vi "Circulos.vi"() -> ()   [LabVIEW 2014]
doc: "Newport Motion Controler\nThis VI test a Group\n\nAndré Romero - 2022\nandretec@ifsc.usp.br"
uses:
  <vilib>/Platform/TimedLoop/XDataNode/timing_clust.ctl
  <vilib>/Platform/TimedLoop/XDataNode/nitl_modes.ctl
  <vilib>/Platform/TimedLoop/XDataNode/wakeup.ctl
  <vilib>/Platform/TimedLoop/XDataNode/XDataNode.xnode
  <userlib>/Newport ESP301/Newport ESP301.lvlib
  <vilib>/Platform/TimedLoop/XDataNode/XDNodeRunTimeDep.lvlib
panel:
  in  "Decceleration (mm/s²)":dbl min=0.0 format="%.6g"
  in  "Acceleration (mm/s²)":dbl min=0.0 format="%.6g"
  in  "coordenada x_centro":dbl format="%#_13g"
  in  "arc sweep angle":dbl=-46.7 format="%#_13g"
  in  "coordenada y_centro":dbl=-5.5 format="%#_13g"
  in  "Stop Button":bool
  out "error out":errorcluster
  out "Y":dbl format="%.2g"
  out "X":dbl=1.0 format="%.2f"
  out "XY Graph":cluster{dbl[], dbl[]}(graph)
  in  "Velocity (mm/s)":dbl=0.05
  # "1o arco"
  # "2o arco"
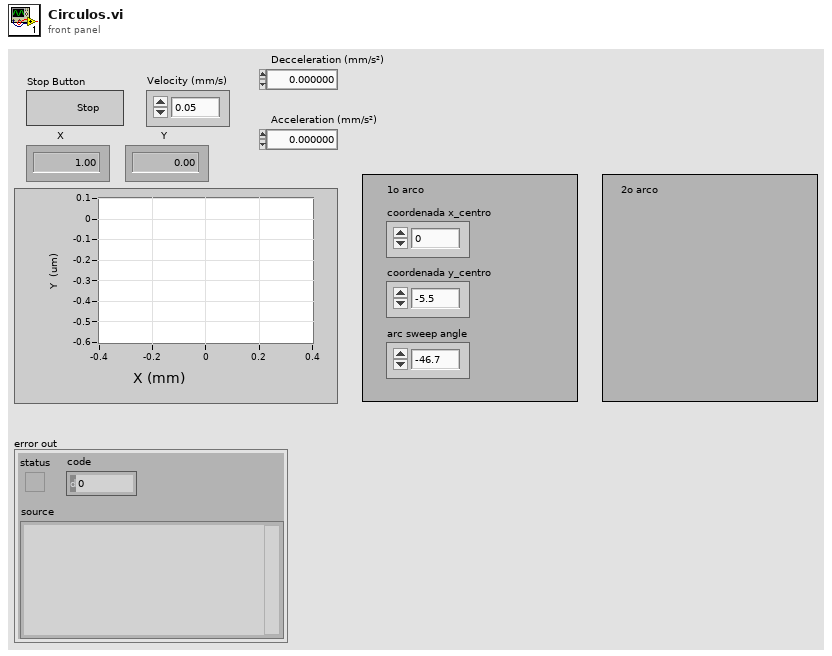
[diagram p1: front panel]
types:
  T1 = typedef "XDNodeRunTimeDep.lvlib/timing_clust.ctl" = cluster{"Expected End [f-1]":u64, "Actual End [f-1]":u64, "Finished Late? [f-1]":bool, "Expected End [i-1]":u64, "Actual End [i-1]":u64, "Finished Late? [i-1]":bool, "Expected Start [i]":u64, "Actual Start [i]":u64, "Expected Start [f]":u64, "Actual Start [f]":u64, "Source Name":string, "Structure Name":string, "Period":i64, "Deadline":i64, "Offset":i64, "Start":i64, "Priority":i32, "Timeout":i32, "Mode":T2, "Wakeup Reason":T3, "Error":errorcluster, "Source Type":string, "Secondary Source Type":string, "Global End Time":u64, "Global Start Time":u64, "Frame Duration":u64, "Iteration Duration":u64, "Assigned CPU":i32, "I/O Scan Engine Mode":u32}
  T2 = typedef "XDNodeRunTimeDep.lvlib/nitl_modes.ctl" = enum32{"No Change", "Process missed periods, maintain original phase", "Discard missed periods, maintain original phase", "Process missed periods, ignore original phase", "Discard missed periods, ignore original phase"}
  T3 = typedef "XDNodeRunTimeDep.lvlib/wakeup.ctl" = enum32{"Normal", "Aborted", "Asynchronous wakeup", "Timing source error", "Timed loop error", "Timeout"}
  T4 = cluster{"coordenada x_centro":dbl, "coordenada y_centro":dbl, "arc sweep angle":dbl}
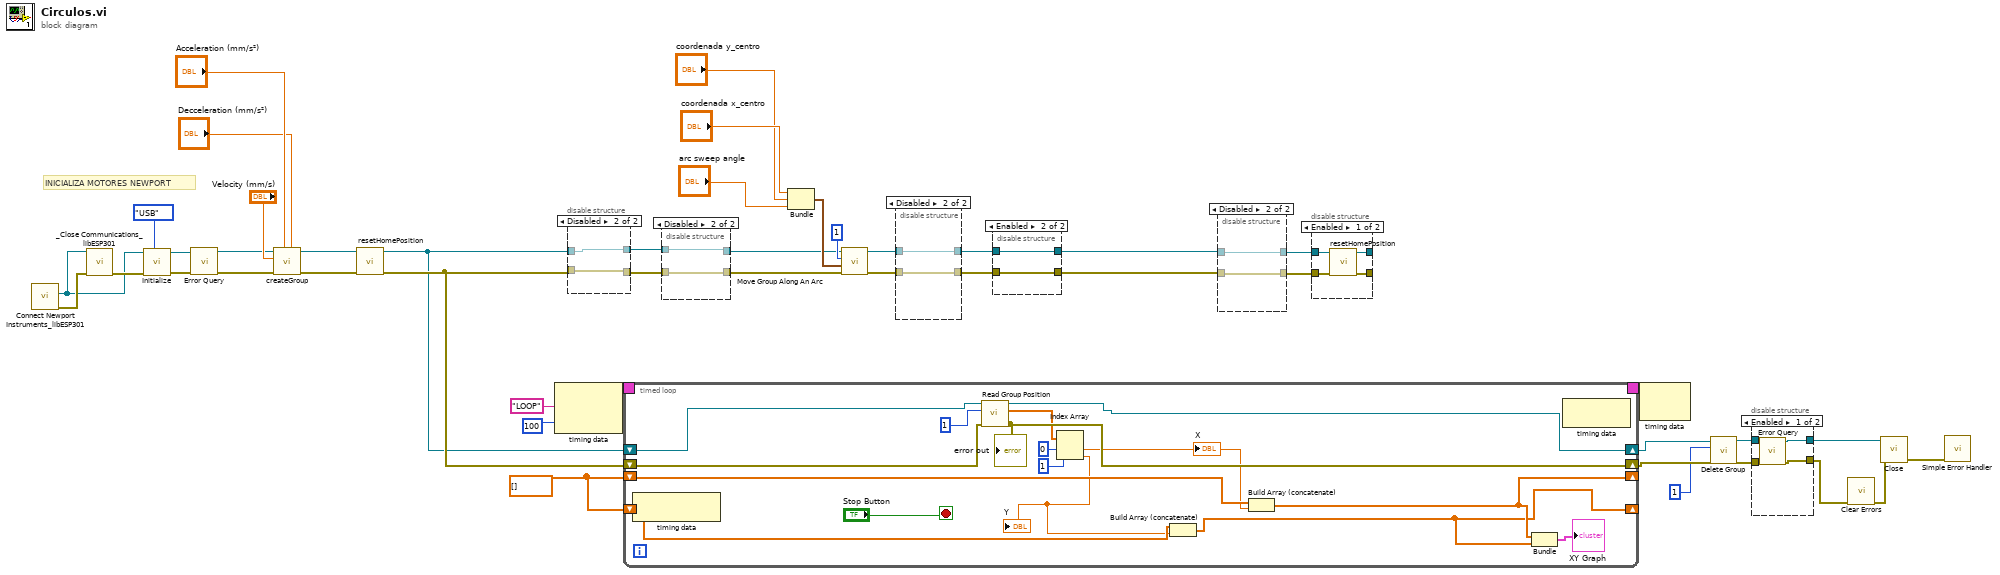
[diagram p0: block diagram]
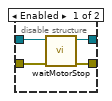
[diagram p2: hidden frame]
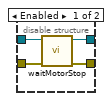
[diagram p3: hidden frame]
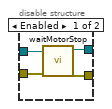
[diagram p4: hidden frame]
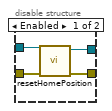
[diagram p6: hidden frame]
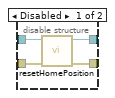
[diagram p7: hidden frame]
diagram:
  w31 = dbl[] []
  # "INICIALIZA MOTORES NEWPORT"
  n1 = call <userlib>:"Connect Newport Instruments_libESP301.vi"() -> ("error (duplicate)"=w44:errorcluster, "VISA resource name (duplicate)"=w43:refnum<visa-resource-name>)  [unwired: 7 in, 3 out]
  n2 = call <userlib>:"_Close Communications_libESP301.vi"("Instrument Channel"=w43, "error in (no error)"=w44) -> ("error out"=w46:errorcluster)  [unwired: 13 in]
  n3 = call <userlib>:"Initialize.vi"("VISA resource name"=w43, "error in (no error)"=w46, "Serial Link (RS232)"=enum16{"RS232", "USB"}."USB") -> ("VISA resource name out"=w42:refnum<visa-resource-name>, "error out"=w41:errorcluster)  [unwired: 6 in]
  n4 = call <userlib>:"Error Query.vi"("error in (no error)"=w41, "VISA resource name"=w42) -> ("error out"=w19:errorcluster, "VISA resource name out"=w20:refnum<visa-resource-name>)  [unwired: 2 in, 2 out]
  n5 = call "createGroup.vi"("Decceleration (0 units/s²)"="Decceleration (mm/s²)", "Acceleration (0 units/s²)"="Acceleration (mm/s²)", "error in (no error)"=w19, "Velocity"="Velocity (mm/s)", "VISA Refnum in"=w20) -> ("error out"=w8:errorcluster, "VISA Refnum out"=w7:refnum<visa-resource-name>)  [unwired: 5 in]
  n6 = call "resetHomePosition.vi"("error in (no error)"=w8, "VISA Refnum in"=w7) -> ("error out"=w2:errorcluster, "VISA Refnum out"=w1:refnum<visa-resource-name>)  [unwired: 8 in]
  n7 = node-c288("LOOP" ("Structure Name"), i64 100 ("Period")) -> (w35:T1)
  n8 = disable-structure shown="Disabled" {
    disable-tunnel: w1 -> [w50 w52]
    disable-tunnel: w2 -> [w49 w51]
    disable-tunnel: [w48 w52] -> w12
    disable-tunnel: [w47 w51] -> w11
    frame Enabled {
      n9 = call "waitMotorStop.vi"("error in (no error)"=w49, "VISA Refnum in"=w50) -> ("error out"=w47:errorcluster, "VISA Refnum out"=w48:refnum<visa-resource-name>)  [unwired: 8 in]
    }
    frame Disabled {
    }
  }
  n10 = timed-loop {
    timing: w35 -> [_]
    timing-out: [_] -> w34
    shift-right: [w63] -> w26
    shift-left: w1 -> [w65]
    shift-right: [w62] -> w25
    shift-left: w2 -> [w64]
    shift-right: [w54] -> _
    shift-left: w31 -> [w68]
    shift-right: [w53] -> _
    shift-left: w31 -> [w67]
    stop <- "Stop Button" stop-if-true
    n11 = node-c288() -> ()  [unwired: 1 in, 1 out]
    n12 = call <userlib>:"Read Group Position.vi"("error in (no error)"=w64, "Group Number (1)"=1, "VISA resource name"=w65) -> ("error out"=w62:errorcluster, "Position (units)"=w59:dbl[], "VISA resource name out"=w63:refnum<visa-resource-name>)  [unwired: 2 in]
    "error out" <- w62
    n13 = Index Array(array=w59, index #1=0 ("index"), index #2=1 ("index")) -> (element #1=w58:dbl, element #2=w57:dbl)
    "Y" <- w57
    "X" <- w58
    n14 = Build Array (concatenate)(w67, w57) -> (w53:dbl[])
    n15 = Build Array (concatenate)(w68, w58) -> (w54:dbl[])
    n16 = Bundle(w54, w53) -> (→"XY Graph":cluster{dbl[], dbl[]})  [unwired: 1 in]
    n17 = node-c288() -> ()  [unwired: 1 in, 1 out]
  }
  n18 = disable-structure shown="Disabled" {
    disable-tunnel: [w74 w76] -> w18
    disable-tunnel: [w73 w75] -> w17
    disable-tunnel: w12 -> [w72 w76]
    disable-tunnel: w11 -> [w71 w75]
    frame Enabled {
      n19 = call "resetHomePosition.vi"("error in (no error)"=w71, "VISA Refnum in"=w72) -> ("error out"=w73:errorcluster, "VISA Refnum out"=w74:refnum<visa-resource-name>)  [unwired: 8 in]
    }
    frame Disabled {
    }
  }
  n20 = Bundle("coordenada x_centro"="coordenada x_centro", "coordenada y_centro"="coordenada y_centro", "arc sweep angle"="arc sweep angle") -> (w36:T4)  [unwired: 1 in]
  n21 = call <userlib>:"Move Group Along An Arc.vi"("error in (no error)"=w17, "Arc  Parameters"=w36, "Group Number (1)"=1, "VISA resource name"=w18) -> ("error out"=w15:errorcluster, "VISA resource name out"=w16:refnum<visa-resource-name>)  [unwired: 2 in]
  n22 = disable-structure shown="Disabled" {
    disable-tunnel: w16 -> [w80 w82]
    disable-tunnel: w15 -> [w79 w81]
    disable-tunnel: [w78 w81] -> w14
    disable-tunnel: [w77 w82] -> w13
    frame Enabled {
      n23 = call "waitMotorStop.vi"("error in (no error)"=w79, "VISA Refnum in"=w80) -> ("error out"=w78:errorcluster, "VISA Refnum out"=w77:refnum<visa-resource-name>)  [unwired: 8 in]
    }
    frame Disabled {
    }
  }
  n24 = disable-structure shown="Enabled" {
    disable-tunnel: [w86 w88] -> w4
    disable-tunnel: [w85 w87] -> w3
    disable-tunnel: w14 -> [w84 w87]
    disable-tunnel: w13 -> [w83 w88]
    frame Disabled {
      n25 = call "resetHomePosition.vi"("error in (no error)"=w84, "VISA Refnum in"=w83) -> ("error out"=w85:errorcluster, "VISA Refnum out"=w86:refnum<visa-resource-name>)  [unwired: 8 in]
    }
    frame Enabled {
    }
  }
  n26 = disable-structure shown="Disabled" {
    disable-tunnel: w3 -> [w92 w93]
    disable-tunnel: w4 -> [w91 w94]
    disable-tunnel: [w90 w94] -> w10
    disable-tunnel: [w89 w93] -> w9
    frame Enabled {
      n27 = call "waitMotorStop.vi"("error in (no error)"=w92, "VISA Refnum in"=w91) -> ("error out"=w89:errorcluster, "VISA Refnum out"=w90:refnum<visa-resource-name>)  [unwired: 8 in]
    }
    frame Disabled {
    }
  }
  n28 = disable-structure shown="Enabled" {
    disable-tunnel: [w98 w100] -> _
    disable-tunnel: [w97 w99] -> _
    disable-tunnel: w10 -> [w96 w100]
    disable-tunnel: w9 -> [w95 w99]
    frame Enabled {
      n29 = call "resetHomePosition.vi"("error in (no error)"=w95, "VISA Refnum in"=w96) -> ("error out"=w97:errorcluster, "VISA Refnum out"=w98:refnum<visa-resource-name>)  [unwired: 8 in]
    }
    frame Disabled {
    }
  }
  n30 = node-c288(w34) -> ()  [unwired: 1 out]
  n31 = call <userlib>:"Delete Group.vi"("error in (no error)"=w25, "Group Number (1)"=1, "VISA resource name"=w26) -> ("error out"=w29:errorcluster, "VISA resource name out"=w30:refnum<visa-resource-name>)  [unwired: 3 in]
  n32 = disable-structure shown="Enabled" {
    disable-tunnel: w30 -> [w104 w106]
    disable-tunnel: w29 -> [w103 w105]
    disable-tunnel: [w102 w106] -> w28
    disable-tunnel: [w101 w105] -> w23
    frame Enabled {
      n33 = call <userlib>:"Error Query.vi"("error in (no error)"=w103, "VISA resource name"=w104) -> ("error out"=w101:errorcluster, "VISA resource name out"=w102:refnum<visa-resource-name>)  [unwired: 2 in, 2 out]
    }
    frame Disabled {
    }
  }
  n34 = call <vilib>:"Clear Errors.vi"("error in (no error)"=w23) -> ("error out"=w22:errorcluster)  [unwired: 5 in, 1 out]
  n35 = call <userlib>:"Close.vi"("error in (no error)"=w22, "VISA resource name"=w28) -> ("error out"=w27:errorcluster)  [unwired: 9 in]
  n36 = call <vilib>:"Simple Error Handler.vi"("error in (no error)"=w27) -> ()  [unwired: 4 in, 5 out]
